vi "Handle Error.vi"(8 "error in (no error)":errorcluster, 11 "MainUI in":refnum<class "MainUI.lvclass">) -> (0 "error out":errorcluster, 2 "stop actor?":bool=TRUE, 3 "MainUI out":refnum<class "MainUI.lvclass">)   [LabVIEW 2019, in "MainUI.lvlib" / "MainUI.lvclass"]
doc: "(<B>Filename</B>: Actor Framework.lvlib:Actor.lvclass:Handle Error.vi)\n\nDefines how the actor handles an error that occurred while processing a message. By default, this method does nothing except stop the actor."
uses:
  MainUI.lvclass
  ModuleAbstract/ModuleAbstract.lvclass
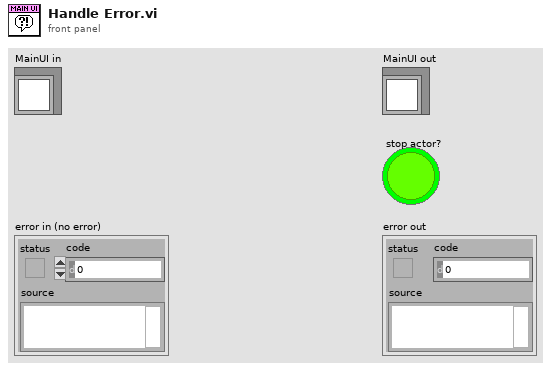
[diagram p1: front panel]
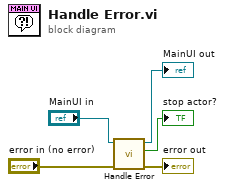
[diagram p0: block diagram]
diagram:
  n1 = call-parent "Handle Error.vi"("error in (no error)"="error in (no error)", "ModuleAbstract in"="MainUI in") -> ("error out"=→"error out":errorcluster, "stop actor?"=→"stop actor?":bool, "ModuleAbstract out"=→"MainUI out":refnum<class "MainUI.lvclass">)  [unwired: 7 in]
